vi "Read-Save DefaultDevice.vi"(6 "Task":enum16{"Save", "Read"}(ring)=enum."Read", 11 "Soundcard":string) -> (0 "Pref Path":path, 3 "Soundcard Out":string)   [LabVIEW 2022 SP3]
panel:
  out "text":string
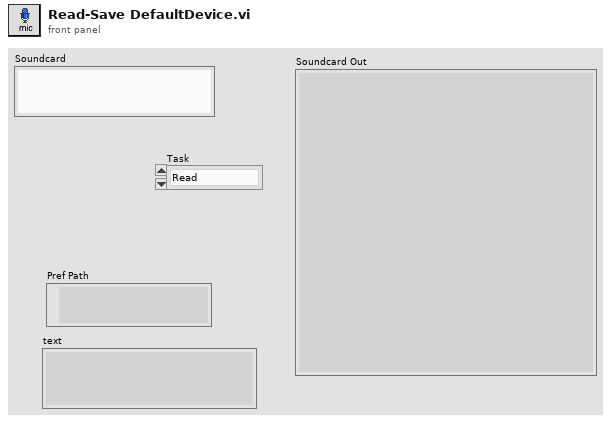
[diagram p1: front panel]
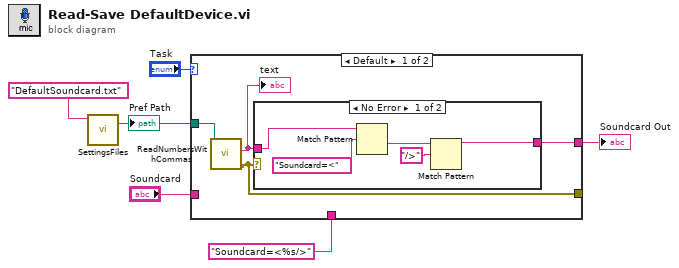
[diagram p0: block diagram]
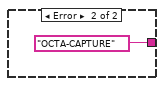
[diagram p2: hidden frame]
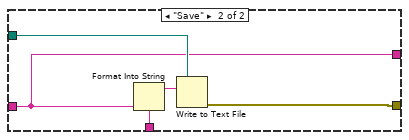
[diagram p3: hidden frame]
diagram:
  n1 = call "SettingsFiles.vi"("settings file name"="DefaultSoundcard.txt" ("name or relative path")) -> ("file path"=w1:path)  [unwired: 9 in, 1 out]
  "Pref Path" <- w1
  n2 = case shown="Default" "Task" {
    tunnel: "Soundcard" -> [_ w18]
    tunnel: w1 -> [w9 w21]
    tunnel: [w7 w19] -> _
    tunnel: [w10 w18] -> w4
    tunnel: "Soundcard=<%s/>" ("format string") -> [_ w17]
    frame Default {
      n3 = call "ReadNumbersWithCommas.vi"("file (use dialog)"=w9) -> ("error out"=w7:errorcluster, "text"=w8:string)  [unwired: 7 in, 2 out]
      "text" <- w8
      n4 = case shown="No Error" w7 {
        tunnel: [w11 "OCTA-CAPTURE" ("Notes")] -> w10
        tunnel: w8 -> [w15 _]
        frame No Error {
          n5 = Match Pattern(string=w15, regular expression="Soundcard=<" ("format string")) -> (after substring=w14:string)  [unwired: 1 in, 3 out]
          n6 = Match Pattern(string=w14, regular expression="/>" ("format string")) -> (before substring=w11:string)  [unwired: 1 in, 3 out]
        }
        frame Error {
        }
      }
    }
    frame "Save" {
      n7 = Format Into String(format string=w17, w18) -> (resulting string=w20:string)  [unwired: 2 in, 1 out]
      n8 = Write to Text File(file (use dialog)=w21, text=w20) -> (error out=w19:errorcluster)  [unwired: 2 in, 2 out]
    }
  }
  "Soundcard Out" <- w4
